vi "SCPI Read Measured Output.vi"(8 "error in (no error)":errorcluster, 11 "VISA resource name":refnum<visa-resource-name>) -> (0 "error out":errorcluster, 1 "Meas Current":dbl format="%.2g", 2 "Meas Voltage":dbl format="%.2g", 3 "VISA resource name out":refnum<visa-resource-name>, 5 "Meas Power":dbl format="%.3g")   [LabVIEW 2021, in "BK Precision 169XB.lvlib"]
doc: "Returns the actual voltage level and actual current level for a desired channel."
uses:
  BK Precision 169XB.lvlib
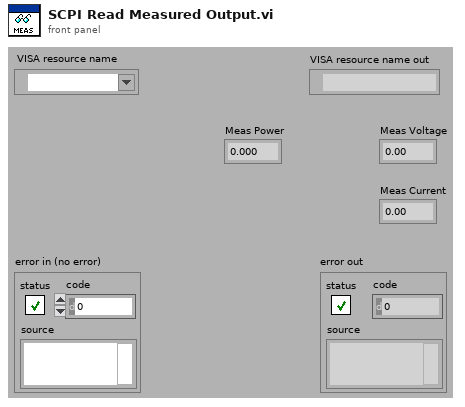
[diagram p1: front panel]
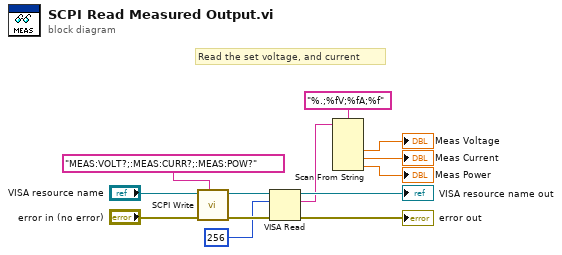
[diagram p0: block diagram]
diagram:
  # "Read the set voltage, and current"
  n1 = call "SCPI Write.vi"("Input String"="MEAS:VOLT?;:MEAS:CURR?;:MEAS:POW?", "error in (no error)"="error in (no error)", "VISA resource name"="VISA resource name") -> ("error out"=w11:errorcluster, "VISA resource name out"=w10:refnum<visa-resource-name>)  [unwired: 7 in]
  n2 = VISA Read(VISA resource name=w10, byte count=u32 256, error in (no error)=w11) -> (VISA resource name out=→"VISA resource name out":refnum<visa-resource-name>, read buffer=w6:string, error out=→"error out":errorcluster)  [unwired: 1 out]
  n3 = Scan From String(format string="%.;%fV;%fA;%f", input string=w6) -> (output 1=→"Meas Voltage":dbl, output 2=→"Meas Current":dbl, output 3=→"Meas Power":dbl)  [unwired: 5 in, 3 out]
